vi "LaserCal-Create Data Header (I-O).vi"(0 "Stimulus":T1, 5 "Response params":T2, 11 "error in (no error)":errorcluster) -> (4 "header":string, 15 "error out":errorcluster)   [LabVIEW 2015]
uses:
  Typedefs/LaserCal-IO Response Params.ctl
  Typedefs/LaserCal-IO Stimulus Params.ctl
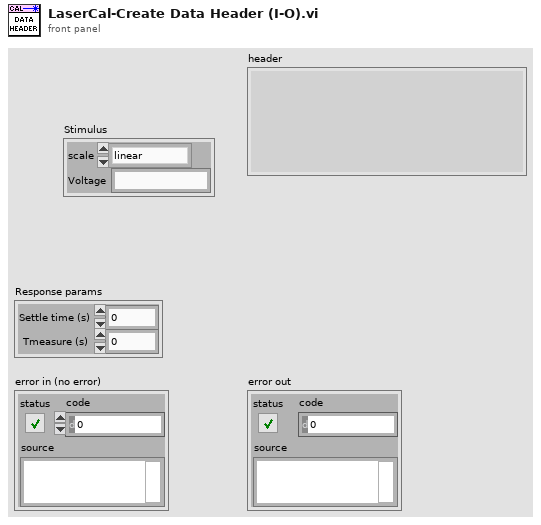
[diagram p1: front panel]
types:
  T1 = typedef "LaserCal-IO Stimulus Params.ctl" = cluster{"scale":enum16{"linear", "dB"}, "Voltage":string}
  T2 = typedef "LaserCal-IO Response Params.ctl" = cluster{"Settle time (s)":dbl, "Tmeasure (s)":dbl}
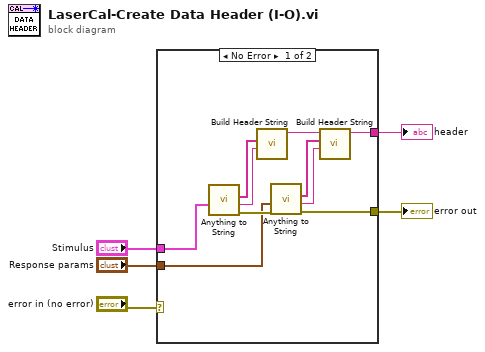
[diagram p0: block diagram]
diagram:
  n1 = case shown="No Error" "error in (no error)" {
    selector: "error in (no error)" -> [_ w16]
    tunnel: [w12 w16] -> w2
    tunnel: "Stimulus" -> [w15 _]
    tunnel: "Response params" -> [w13 _]
    tunnel: [w6 _] -> w5
    frame No Error {
      n2 = call "Anything to String.vi"("Anything"=w15) -> ("Error Out"=w14:errorcluster, "Section"=w10:string, "Strings[]"=w11:string[])  [unwired: 8 in]
      n3 = call "Build Header String.vi"("Section"=w10, "Strings[]"=w11) -> ("Header out"=w9:string)  [unwired: 9 in]
      n4 = call "Anything to String.vi"("Error In"=w14, "Anything"=w13) -> ("Error Out"=w12:errorcluster, "Section"=w7:string, "Strings[]"=w8:string[])  [unwired: 7 in]
      n5 = call "Build Header String.vi"("Section"=w7, "Strings[]"=w8, "Header in"=w9) -> ("Header out"=w6:string)  [unwired: 8 in]
    }
    frame Error {
    }
  }
  "header" <- w5
  "error out" <- w2
